vi "Userlist Message Callback.vi"(7 "Owner":refnum<class>, 11 "Message":refnum<class "Message.lvclass">) -> (0 "error out":errorcluster)   [LabVIEW 2020, in "LV Chat Client.lvclass"]
uses:
  LV Chat Client.lvclass
  Stream-Simple-Msg/Message/Message.lvclass
  LV Chat Client.lvclass/LV Chat Client.ctl
  9460544c-6bf9-4dc1-88bc-113ddb7eadc4.vi
  Stream-Simple-Msg/Message/Get Data.vi
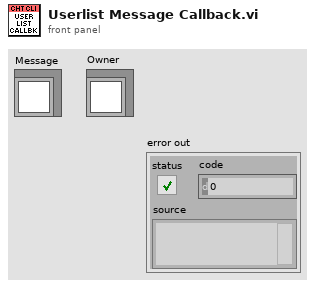
[diagram p1: front panel]
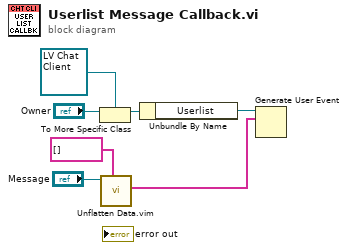
[diagram p0: block diagram]
diagram:
  n1 = To More Specific Class(target class=refnum<class "LV Chat Client.lvclass"> refnum ("LV Chat Client.lvclass"), reference="Owner") -> (specific class reference=w3:refnum<class "LV Chat Client.lvclass">)  [unwired: 1 in, 1 out]
  n2 = call "Unflatten Data.vim"("Data Type"=string[] [], "Message in"="Message") -> ("Unflattened Data"=w1:string[])  [unwired: 7 in, 2 out]
  n3 = Unbundle By Name(w3) -> ("Userlist"=w2:refnum<user-event>)
  n4 = Generate User Event(user event=w2, event data cluster=w1) -> ()  [unwired: 2 in, 2 out]
